vi "Test.vi"   [LabVIEW 2016]
uses:
  <vilib>/NXT/Hardware/Plugins/Tetrix DC Motor/TetrixDCMotorAddress.ctl
  <vilib>/NXT/LegoClasses/BrickReference/BrickReference.lvclass
  <vilib>/NXT/Subs/LVHSConnector.ctl
  <vilib>/NXT/NXTIO Xnodes/NXTIONodeSubVIs/TETRIX IO Move DC Motors.vi
  <vilib>/NXT/NXTIO Xnodes/NXTIOXNode/NXTIO.xnode
  <vilib>/NXT/NXTIO Xnodes/AddressXNode/NXTIOAddress.xnode
  Program1.lvrbt
  <vilib>/NXT/Dual Mode Library/Waits/Wait_Num.vi
  <vilib>/NXT/Subs/ColorSensorColors.ctl
  <vilib>/NXT/Block Support/NXT_InputPort.ctl
  <vilib>/NXT/Dual Mode Library/Sensors/EV3_Color_Color.vi
types:
  T1 = typedef "TetrixDCMotorAddress.ctl" = i32
  T2 = typedef "LVHSConnector.ctl" = refnum<class "BrickReference.lvclass">
  T3 = cluster{"TetrixDCMotor":T1, "TetrixDCMotor 2":T1}
  T4 = typedef "NXT_InputPort.ctl" = u32
  T5 = typedef "ColorSensorColors.ctl" = enum16{"No Color", "Black", "Blue", "Green", "Yellow", "Red", "White", "Brown"}
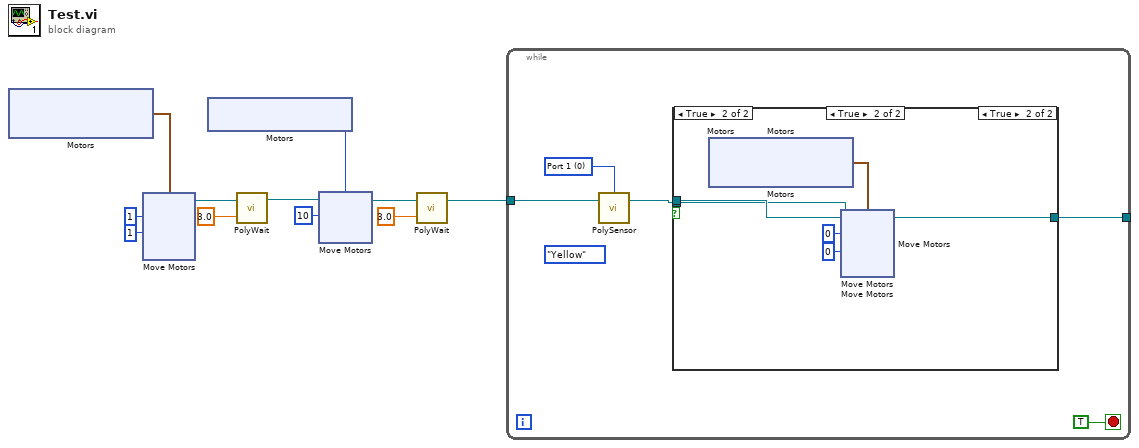
[diagram p0: block diagram]
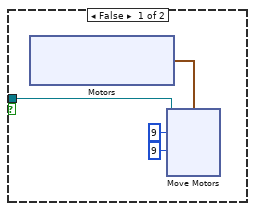
[diagram p2: hidden frame]
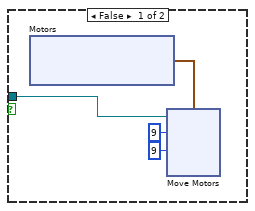
[diagram p3: hidden frame]
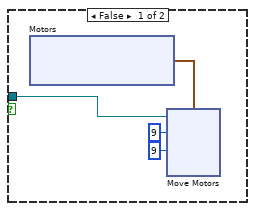
[diagram p4: hidden frame]
diagram:
  n1 = xnode "Motors"() -> ("Motor"=w11:cluster{"TetrixDCMotor":T1, "TetrixDCMotor":T1})
  n2 = xnode "Move Motors"("Power/Speed 2"=i8 1, "Power/Speed 1"=i8 1, "Motors"=w11) -> ("NXT/EV3"=w8:T2)  [unwired: 1 in]
  n3 = xnode "Motors"() -> ("Motor"=w4:T1)
  n4 = call-poly <vilib>:"PolyWait.vi"("Time (1 sec)"=sgl 3.0, "NXT/EV3"=w8) -> ("NXT/EV3"=w6:T2)  [unwired: 2 in]
  n5 = xnode "Move Motors"("Power/Speed 1"=i8 10, "Motors"=w4, "NXT/EV3"=w6) -> ("NXT/EV3"=w3:T2)
  n6 = call-poly <vilib>:"PolyWait.vi"("Time (1 sec)"=sgl 3.0, "NXT/EV3"=w3) -> ("NXT/EV3"=w1:T2)  [unwired: 2 in]
  n7 = while {
    tunnel: w1 -> [w16]
    tunnel: [w13] -> _
    stop <- TRUE stop-if-true
    w15 = T4 0 items=["Port 1", "Port 2", "Port 3", "Port 4"] ("Port (Port 1)")
    (unwired) ColorSensorColors."Yellow" ("Detected Color")
    n8 = call-poly <vilib>:"PolySensor.vi"("NXT/EV3"=w16, "Port (Port 1)"=w15) -> ("NXT/EV3"=w12:T2)  [unwired: 1 in, 1 out]
    n9 = case shown="True" {
      selector: _ -> [_ _]
      tunnel: [_ w31] -> _
      tunnel: w12 -> [w17 w30]
      frame False {
        n10 = xnode "Motors"() -> ("Motor"=w20:cluster{"TetrixDCMotor":T1, "TetrixDCMotor":T1})
        n11 = xnode "Move Motors"("Power/Speed 2"=i8 9, "Power/Speed 1"=i8 9, "Motors"=w20, "NXT/EV3"=w17) -> ()  [unwired: 1 out]
      }
      frame True {
        n12 = xnode "Motors"() -> ("Motor"=w34:cluster{"TetrixDCMotor":T1, "TetrixDCMotor":T1})
        n13 = xnode "Move Motors"("Power/Speed 2"=i8 0, "Power/Speed 1"=i8 0, "Motors"=w34, "NXT/EV3"=w30) -> ("NXT/EV3"=w31:T2)
      }
    }
    n14 = case shown="True" {
      selector: _ -> [_ _]
      tunnel: _ -> [w46 w57]
      tunnel: [_ w58] -> _
      frame False {
        n15 = xnode "Motors"() -> ("Motor"=w47:cluster{"TetrixDCMotor":T1, "TetrixDCMotor":T1})
        n16 = xnode "Move Motors"("Power/Speed 2"=i8 9, "Power/Speed 1"=i8 9, "Motors"=w47, "NXT/EV3"=w46) -> ()  [unwired: 1 out]
      }
      frame True {
        n17 = xnode "Motors"() -> ("Motor"=w61:cluster{"TetrixDCMotor":T1, "TetrixDCMotor":T1})
        n18 = xnode "Move Motors"("Power/Speed 2"=i8 0, "Power/Speed 1"=i8 0, "Motors"=w61, "NXT/EV3"=w57) -> ("NXT/EV3"=w58:T2)
      }
    }
    n19 = case shown="True" {
      selector: _ -> [_ _]
      tunnel: _ -> [w73 w84]
      tunnel: [_ w85] -> w13
      frame False {
        n20 = xnode "Motors"() -> ("Motor"=w74:cluster{"TetrixDCMotor":T1, "TetrixDCMotor":T1})
        n21 = xnode "Move Motors"("Power/Speed 2"=i8 9, "Power/Speed 1"=i8 9, "Motors"=w74, "NXT/EV3"=w73) -> ()  [unwired: 1 out]
      }
      frame True {
        n22 = xnode "Motors"() -> ("Motor"=w88:cluster{"TetrixDCMotor":T1, "TetrixDCMotor":T1})
        n23 = xnode "Move Motors"("Power/Speed 2"=i8 0, "Power/Speed 1"=i8 0, "Motors"=w88, "NXT/EV3"=w84) -> ("NXT/EV3"=w85:T2)
      }
    }
  }
